vi "Write Subdiagrams.vi"(8 "error in (no error)":errorcluster, 10 "Subdiagrams":map{string, T1}(c390), 11 "Structure in":refnum<class "Structure.lvclass">) -> (0 "error out":errorcluster, 3 "Structure out":refnum<class "Structure.lvclass">)   [LabVIEW 2025, in "Structure.lvclass"]
uses:
  Structure.lvclass
  Controls/Subdiagram.ctl
  Structure.lvclass/Structure.ctl
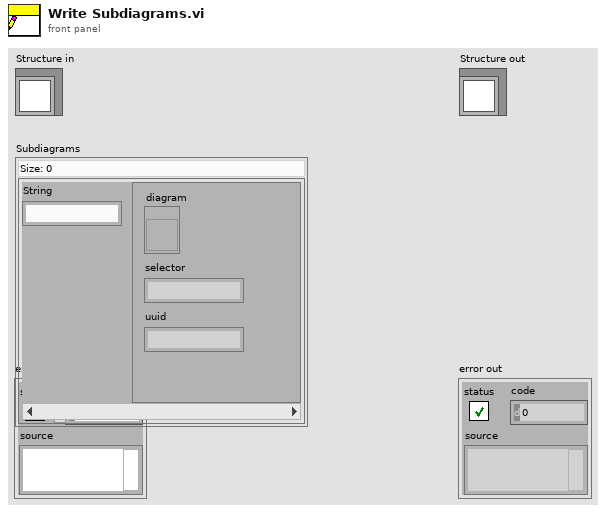
[diagram p1: front panel]
types:
  T1 = typedef "Subdiagram.ctl" = cluster{"diagram":refnum<vi>, "selector":string, "uuid":string}
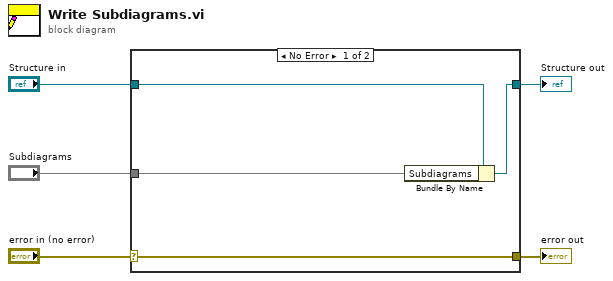
[diagram p0: block diagram]
diagram:
  n1 = case shown="No Error" "error in (no error)" {
    selector: "error in (no error)" -> [w9 w10]
    tunnel: [w9 w10] -> w4
    tunnel: [w7 w11] -> w2
    tunnel: "Structure in" -> [w8 w11]
    tunnel: "Subdiagrams" -> [w6 _]
    frame No Error {
      n2 = Bundle By Name(cluster=w8, "Subdiagrams"=w6) -> (w7:refnum<class "Structure.lvclass">)
    }
    frame Error {
    }
  }
  "error out" <- w4
  "Structure out" <- w2
